vi "tsapp_stop_logging.vi"(8 "error in (no error)":errorcluster, 11 "Path":path) -> (0 "error out":errorcluster, 2 "retuen":i32, 3 "Path output":path)   [LabVIEW 2014]
doc: "Function Introduction\nStop message recording\nCall location\nThis function needs to be used in conjunction with tsapp_dart-logging to stop message recording, and the message will be saved\nSave as the corresponding BLF file.\ninput parameter \nnothing\nReturn value==0: Successful execution\nOther values: Query error codes"
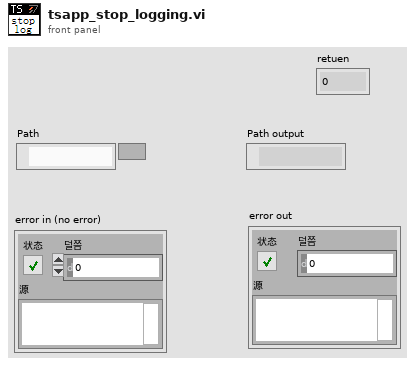
[diagram p1: front panel]
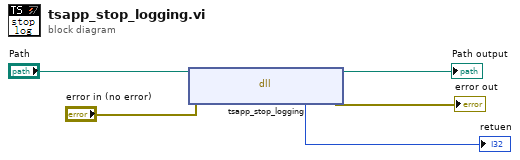
[diagram p0: block diagram]
diagram:
  n1 = dll-call lib="D:/Program Files (x86)/TOSUN/TSMaster/bin/TSMaster.dll" fn="tsapp_stop_logging"(path in="Path", error in="error in (no error)") -> (path out=→"Path output":path, error out=→"error out":errorcluster, "rerurn"=→"retuen":i32)  [unwired: 1 in]
